vi "Periodic Tasks.vi"() -> ()   [LabVIEW 2012]
doc: "This VI runs in parallel to other tasks. It can contain as many user-defined periodic loops as you need. These can carry out PID or other sorts of timed response."
uses:
  <vilib>/Rock Robotics/SystemInterfaces/Utilities/FPGA_UtilitiesLED Source.ctl
  <vilib>/Rock Robotics/SystemInterfaces/Utilities/FPGA_UtilitiesLED State.ctl
  Robot Global Data.vi
panel:
  in  "Shoot Deadband":dbl=0.05
  out "Angular Rate":dbl
  out "Angle":dbl
  out "Rate":dbl
  out "Direction":bool
  out "Distance":dbl
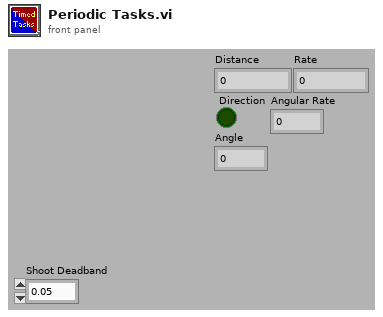
[diagram p1: front panel]
types:
  T1 = typedef "FPGA_UtilitiesLED State.ctl" = enum16{"Off", "On", "Toggle"}
  T2 = typedef "FPGA_UtilitiesLED Source.ctl" = enum16{"User LED", "FPGA LED"}
  T3 = cluster{"ShootTrackEnable":bool, "ShootStartWheels":bool, "ShootIndexerEnable":bool, "ShootCase":dbl, "ShootPOTElev":dbl, "ShootManualElev":dbl, "IndexerSpeed":dbl, "Wheel Spd F":dbl, "Deadband":dbl, "ShootTargetInfo":cluster{"X Coord":dbl, "Y Coord":dbl, "Distance":dbl}, "ShootConstElev":cluster{"1":dbl, "2":dbl, "3":dbl, "4":dbl, "Ground":dbl}, "ShootRollerSpd":dbl, "ShootFlipperPE":bool, "ShootConstFlipper":cluster{"Down":dbl, "Up":dbl}, "Wheel Spd B":dbl}
  T4 = cluster{"ClimbManualExt":dbl, "ClimbManualDep":dbl, "ClimbRetEnable":bool, "ClimbPOTDep":dbl, "ClimbConst":cluster{"ClimbConstDep":dbl, "ClimbConstFold":dbl, "ClimbConstExt":dbl, "ClimbConstRet":dbl}, "ClimbPOTExt":dbl, "ClimbExtEnable":bool, "ClimbLimit":bool, "ClimbFoldEnable":bool, "ClimbDepEnable":bool, "ClimbCase":dbl}
  T5 = typedef "WPI_GyroDevRef.ctl" = cluster{"DevStatus":errorcluster, "Analog Module":T6, "Analog Channel":T7, "Offset":dbl, "Gain (VoltsPerDegree/Second)":dbl}
  T6 = typedef "FPGA_TypedefAnalogModule.ctl" = enum16{"Analog Module 1", "Analog Module 2"}
  T7 = typedef "FPGA_AIChannel.ctl" = enum8{"AI 1", "AI 2", "AI 3", "AI 4", "AI 5", "AI 6", "AI 7", "AI 8", "Invalid"}
  T8 = typedef "WPI_EncoderDevRef.ctl" = cluster{"DevStatus":errorcluster, "EncoderIndex":T9, "CounterIndex":T10, "DistancePerCount":dbl, "Decoding Type":T11}
  T9 = typedef "FPGA_EncoderIdx.ctl" = enum8{"Enc 0", "Enc 1", "Enc 2", "Enc 3", "Invalid"}
  T10 = typedef "FPGA_CounterCtrSystemIndex.ctl" = enum8{"Ctr 0", "Ctr 1", "Ctr 2", "Ctr 3", "Ctr 4", "Ctr 5", "Ctr 6", "Ctr 7", "Invalid"}
  T11 = typedef "WPI_EncoderType.ctl" = enum16{"1x", "2x", "4x"}
  T12 = typedef "WPI_DigitalInputDevRef.ctl" = cluster{"DevStatus":errorcluster, "DIO Channel":T13, "Digital Module":T14}
  T13 = typedef "FPGA_DIOChannel.ctl" = enum8{"DIO 1", "DIO 2", "DIO 3", "DIO 4", "DIO 5", "DIO 6", "DIO 7", "DIO 8", "DIO 9", "DIO 10", "DIO 11", "DIO 12", "DIO 13", "DIO 14", "Invalid"}
  T14 = typedef "FPGA_TypedefDigitalModule.ctl" = enum16{"Digital Module 1", "Digital Module 2"}
  T15 = typedef "WPI_AnalogChannelDevRef.ctl" = cluster{"DevStatus":errorcluster, "Analog Module":T6, "Analog Channel":T7}
  T16 = cluster{"Ground":dbl, "1":dbl, "2":dbl, "3":dbl, "4":dbl}
  T17 = cluster{"ShootOutIndexer":dbl, "ShootOutElev":dbl, "ShootCase":dbl, "ShootOutWheelF":dbl, "ShootOutWheelB":dbl, "ShootOutRollers":dbl, "ShootOutFlipper":dbl}
  T18 = cluster{"ClimbConstDep":dbl, "ClimbConstFold":dbl, "ClimbConstExt":dbl, "ClimbConstRet":dbl}
  T19 = cluster{"ClimbOutDep":dbl, "ClimbOutExt":dbl, "ClimbOutCase":i32}
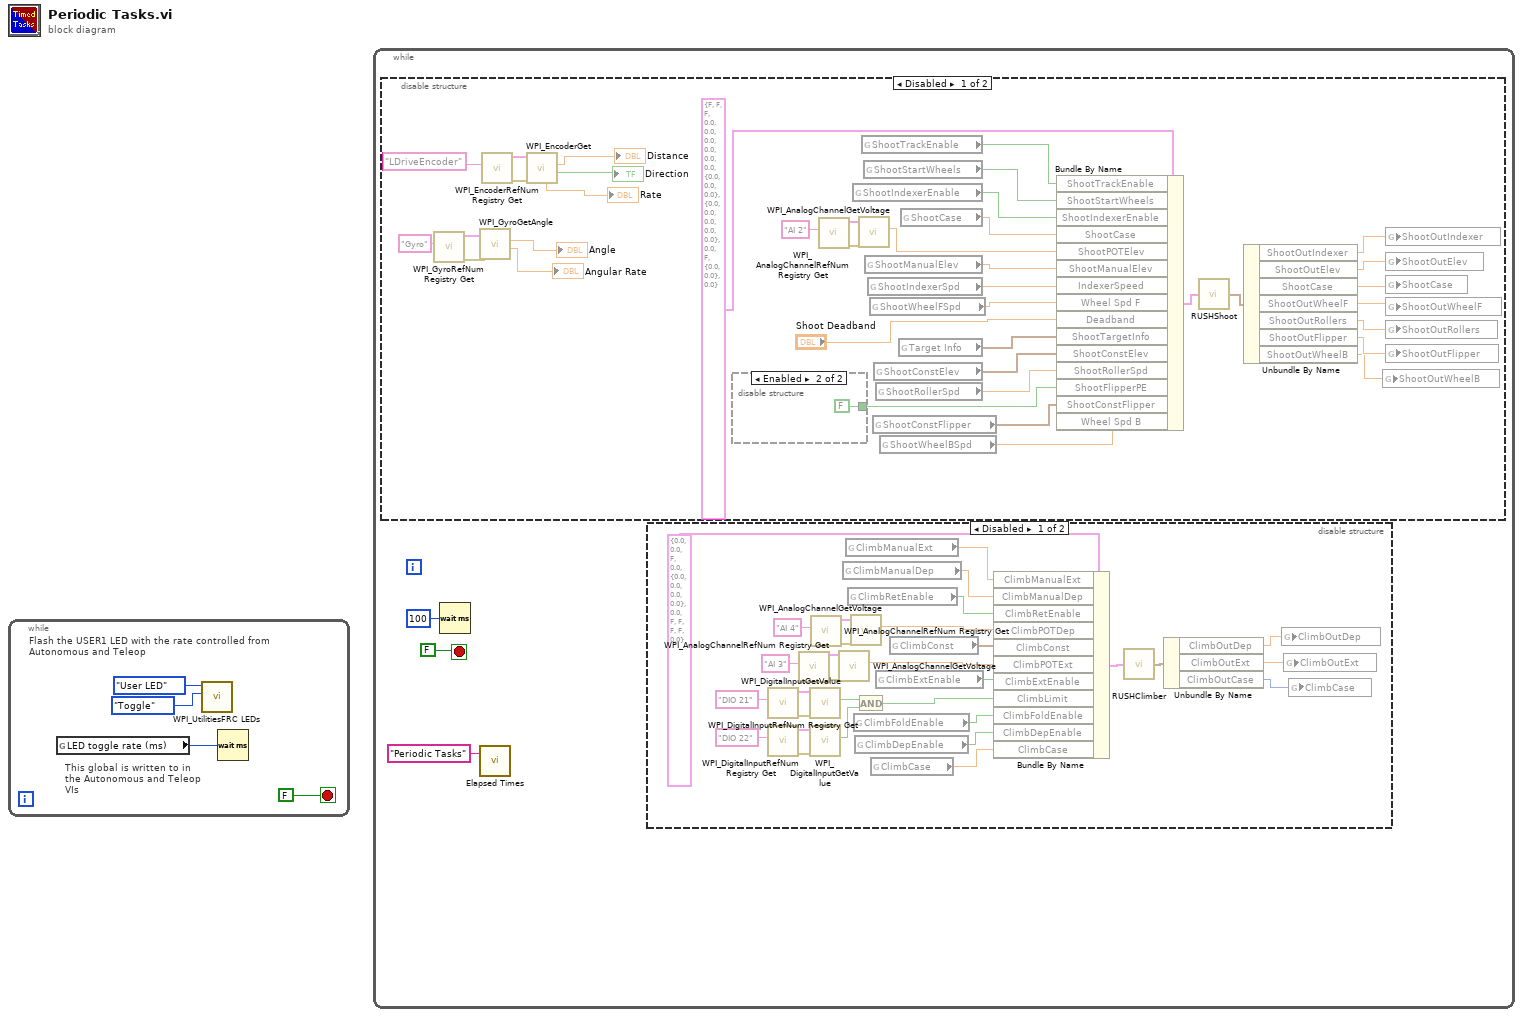
[diagram p0: block diagram]
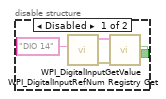
[diagram p2: hidden frame]
diagram:
  n1 = while {
    stop <- FALSE stop-if-true
    # "This global is written to in the Autonomous and Teleop VIs"
    # "Flash the USER1 LED with the rate controlled from Autonomous and Teleop"
    n2 = global read "Robot Global Data.vi" "LED toggle rate (ms)"() -> (w1:u32)
    n3 = call <vilib>:"WPI_UtilitiesFRC LEDs.vi"("State"=FPGA_UtilitiesLED_State."Toggle", "LED Type"=FPGA_UtilitiesLED_Source."User LED") -> ()  [unwired: 1 in, 9 out]
    n4 = Wait (ms)(milliseconds to wait=w1) -> ()  [unwired: 1 out]
  }
  n5 = while {
    stop <- FALSE stop-if-true
    n6 = disable-structure shown="Disabled" {
      frame Disabled {
        n7 = call <vilib>:"WPI_GyroRefNum Registry Get.vi"("refnum name"="Gyro") -> ("error out"=w44:errorcluster, "GyroDevRef"=w43:T5)  [unwired: 9 in]
        n8 = call <vilib>:"WPI_GyroGetAngle.vi"("error in (no error)"=w44, "GyroDevRef"=w43) -> ("Angular Rate"=→"Angular Rate":dbl, "Angle"=→"Angle":dbl)  [unwired: 6 in, 2 out]
        n9 = call <vilib>:"WPI_EncoderRefNum Registry Get.vi"("refnum name"="LDriveEncoder") -> ("error out"=w46:errorcluster, "EncoderDevRef"=w45:T8)  [unwired: 9 in]
        n10 = call <vilib>:"WPI_EncoderGet.vi"("error in (no error)"=w46, "EncoderDevRef"=w45) -> ("Direction"=→"Direction":bool, "Distance"=→"Distance":dbl, "Rate"=→"Rate":dbl)  [unwired: 4 in, 3 out]
        n11 = disable-structure shown="Enabled" {
          disable-tunnel: [w47 FALSE ("Value")] -> w13
          frame Disabled {
            n12 = call <vilib>:"WPI_DigitalInputRefNum Registry Get.vi"("refnum name"="DIO 14") -> ("error out"=w50:errorcluster, "DigitalInputDevRef"=w49:T12)  [unwired: 9 in]
            n13 = call <vilib>:"WPI_DigitalInputGetValue.vi"("error in (no error)"=w50, "DigitalInputDevRef"=w49) -> ("Value"=w47:bool)  [unwired: 7 in, 2 out]
          }
          frame Enabled {
          }
        }
        n14 = call <vilib>:"WPI_AnalogChannelRefNum Registry Get.vi"("refnum name"="AI 2") -> ("error out"=w16:errorcluster, "AIDeviceRef"=w15:T15)  [unwired: 9 in]
        n15 = global read "Robot Global Data.vi" "ShootIndexerEnable"() -> (w27:bool)
        n16 = call <vilib>:"WPI_AnalogChannelGetVoltage.vi"("error in (no error)"=w16, "AIDeviceRef"=w15) -> ("Voltage"=w14:dbl)  [unwired: 7 in, 2 out]
        n17 = global read "Robot Global Data.vi" "ShootTrackEnable"() -> (w29:bool)
        n18 = global read "Robot Global Data.vi" "ShootStartWheels"() -> (w28:bool)
        n19 = global read "Robot Global Data.vi" "ShootManualElev"() -> (w26:dbl)
        n20 = global read "Robot Global Data.vi" "ShootIndexerSpd"() -> (w34:dbl)
        n21 = global read "Robot Global Data.vi" "ShootWheelFSpd"() -> (w33:dbl)
        n22 = global read "Robot Global Data.vi" "ShootConstFlipper"() -> (w30:cluster{"Down":dbl, "Up":dbl})
        n23 = global read "Robot Global Data.vi" "ShootConstElev"() -> (w31:T16)
        n24 = global read "Robot Global Data.vi" "ShootRollerSpd"() -> (w25:dbl)
        n25 = global read "Robot Global Data.vi" "ShootWheelBSpd"() -> (w9:dbl)
        n26 = global read "Robot Global Data.vi" "Target Info"() -> (w32:cluster{"X":dbl, "Y":dbl, "Distance (ft)":dbl})
        n27 = global read "Robot Global Data.vi" "ShootCase"() -> (w35:dbl)
        n28 = Bundle By Name(cluster=T3 {"ShootTrackEnable"=FALSE, "ShootStartWheels"=FALSE, "ShootIndexerEnable"=FALSE, "ShootCase"=0.0, "ShootPOTElev"=0.0, "ShootManualElev"=0.0, "IndexerSpeed"=0.0, "Wheel Spd F"=0.0, "Deadband"=0.0, "ShootTargetInfo"={"X Coord"=0.0, "Y Coord"=0.0, "Distance"=0.0}, "ShootConstElev"={"1"=0.0, "2"=0.0, "3"=0.0, "4"=0.0, "Ground"=0.0}, "ShootRollerSpd"=0.0, "ShootFlipperPE"=FALSE, "ShootConstFlipper"={"Down"=0.0, "Up"=0.0}, "Wheel Spd B"=0.0} ("In Cluster"), "ShootTrackEnable"=w29, "ShootStartWheels"=w28, "ShootIndexerEnable"=w27, "ShootCase"=w35, "ShootPOTElev"=w14, "ShootManualElev"=w26, "IndexerSpeed"=w34, "Wheel Spd F"=w33, "Deadband"="Shoot Deadband", "ShootTargetInfo"=w32, "ShootConstElev"=w31, "ShootRollerSpd"=w25, "ShootFlipperPE"=w13, "ShootConstFlipper"=w30, "Wheel Spd B"=w9) -> (w10:T3)
        n29 = call "RUSHShoot.vi"("In Cluster"=w10) -> ("Out Cluster"=w24:T17)
        n30 = Unbundle By Name(w24) -> ("ShootOutIndexer"=w21:dbl, "ShootOutElev"=w22:dbl, "ShootCase"=w23:dbl, "ShootOutWheelF"=w20:dbl, "ShootOutRollers"=w19:dbl, "ShootOutFlipper"=w18:dbl, "ShootOutWheelB"=w8:dbl)
        n31 = global write "Robot Global Data.vi" "ShootOutWheelB"(w8) -> ()
        n32 = global write "Robot Global Data.vi" "ShootOutIndexer"(w21) -> ()
        n33 = global write "Robot Global Data.vi" "ShootOutElev"(w22) -> ()
        n34 = global write "Robot Global Data.vi" "ShootCase"(w23) -> ()
        n35 = global write "Robot Global Data.vi" "ShootOutWheelF"(w20) -> ()
        n36 = global write "Robot Global Data.vi" "ShootOutRollers"(w19) -> ()
        n37 = global write "Robot Global Data.vi" "ShootOutFlipper"(w18) -> ()
      }
      frame Enabled {
      }
    }
    n38 = Wait (ms)(milliseconds to wait=u32 100) -> ()  [unwired: 1 out]
    n39 = call "Elapsed Times.vi"("Call Name"="Periodic Tasks") -> ()  [unwired: 2 in, 1 out]
    n40 = disable-structure shown="Disabled" {
      frame Disabled {
        n41 = call <vilib>:"WPI_DigitalInputRefNum Registry Get.vi"("refnum name"="DIO 21") -> ("error out"=w77:errorcluster, "DigitalInputDevRef"=w78:T12)  [unwired: 9 in]
        n42 = call <vilib>:"WPI_DigitalInputRefNum Registry Get.vi"("refnum name"="DIO 22") -> ("error out"=w76:errorcluster, "DigitalInputDevRef"=w75:T12)  [unwired: 9 in]
        n43 = call <vilib>:"WPI_AnalogChannelRefNum Registry Get.vi"("refnum name"="AI 3") -> ("error out"=w65:errorcluster, "AIDeviceRef"=w64:T15)  [unwired: 9 in]
        n44 = call <vilib>:"WPI_DigitalInputGetValue.vi"("error in (no error)"=w77, "DigitalInputDevRef"=w78) -> ("Value"=w72:bool)  [unwired: 7 in, 2 out]
        n45 = call <vilib>:"WPI_DigitalInputGetValue.vi"("error in (no error)"=w76, "DigitalInputDevRef"=w75) -> ("Value"=w73:bool)  [unwired: 7 in, 2 out]
        n46 = call <vilib>:"WPI_AnalogChannelRefNum Registry Get.vi"("refnum name"="AI 4") -> ("error out"=w70:errorcluster, "AIDeviceRef"=w68:T15)  [unwired: 9 in]
        n47 = call <vilib>:"WPI_AnalogChannelGetVoltage.vi"("error in (no error)"=w65, "AIDeviceRef"=w64) -> ("Voltage"=w63:dbl)  [unwired: 7 in, 2 out]
        n48 = global read "Robot Global Data.vi" "ClimbManualDep"() -> (w61:dbl)
        n49 = global read "Robot Global Data.vi" "ClimbManualExt"() -> (w62:dbl)
        n50 = global read "Robot Global Data.vi" "ClimbRetEnable"() -> (w60:bool)
        n51 = call <vilib>:"WPI_AnalogChannelGetVoltage.vi"("error in (no error)"=w70, "AIDeviceRef"=w68) -> ("Voltage"=w67:dbl)  [unwired: 7 in, 2 out]
        n52 = global read "Robot Global Data.vi" "ClimbFoldEnable"() -> (w57:bool)
        n53 = global read "Robot Global Data.vi" "ClimbDepEnable"() -> (w56:bool)
        n54 = And(x=w72, y=w73) -> (x .and. y?=w71:bool)
        n55 = global read "Robot Global Data.vi" "ClimbCase"() -> (w55:dbl)
        n56 = global read "Robot Global Data.vi" "ClimbExtEnable"() -> (w58:bool)
        n57 = global read "Robot Global Data.vi" "ClimbConst"() -> (w59:T18)
        n58 = Bundle By Name(cluster=T4 {"ClimbManualExt"=0.0, "ClimbManualDep"=0.0, "ClimbRetEnable"=FALSE, "ClimbPOTDep"=0.0, "ClimbConst"={"ClimbConstDep"=0.0, "ClimbConstFold"=0.0, "ClimbConstExt"=0.0, "ClimbConstRet"=0.0}, "ClimbPOTExt"=0.0, "ClimbExtEnable"=FALSE, "ClimbLimit"=FALSE, "ClimbFoldEnable"=FALSE, "ClimbDepEnable"=FALSE, "ClimbCase"=0.0} ("In Cluster 2"), "ClimbManualExt"=w62, "ClimbManualDep"=w61, "ClimbRetEnable"=w60, "ClimbPOTDep"=w67, "ClimbConst"=w59, "ClimbPOTExt"=w63, "ClimbExtEnable"=w58, "ClimbLimit"=w71, "ClimbFoldEnable"=w57, "ClimbDepEnable"=w56, "ClimbCase"=w55) -> (w81:T4)
        n59 = call "RUSHClimber.vi"("In Cluster"=w81) -> ("Out Cluster"=w80:T19)
        n60 = Unbundle By Name(w80) -> ("ClimbOutDep"=w52:dbl, "ClimbOutExt"=w53:dbl, "ClimbOutCase"=w54:i32)
        n61 = global write "Robot Global Data.vi" "ClimbOutDep"(w52) -> ()
        n62 = global write "Robot Global Data.vi" "ClimbOutExt"(w53) -> ()
        n63 = global write "Robot Global Data.vi" "ClimbCase"(w54) -> ()
      }
      frame Enabled {
      }
    }
  }
